vi "test SSL Client Invalid Hostname.vi"(8 "error in (no error)":errorcluster, 11 "TestCase in":refnum<class "test SSL Client.lvclass">) -> (0 "error out":errorcluster, 3 "TestCase out":refnum<class "test SSL Client.lvclass">)   [LabVIEW 2013, in "test SSL Client.lvclass"]
uses:
  test SSL Client.lvclass
  <vilib>/addons/_JKI Toolkits/VI Tester/TestCase.llb/TestCase.lvclass
  SSL_Lib/BIO/BIO.lvclass
  <vilib>/Utility/error.llb/DialogType.ctl
  SSL_Lib/SSL-Context/SSL-Context.lvclass
  SSL_Lib/SSL/SSL.lvclass
  SSL_Lib/SSL/SSL_Mode.ctl
  suite SSL Client/suite SSL Client/SSL Context.vi
  suite SSL Client/suite SSL Client/suite SSL Client.lvclass
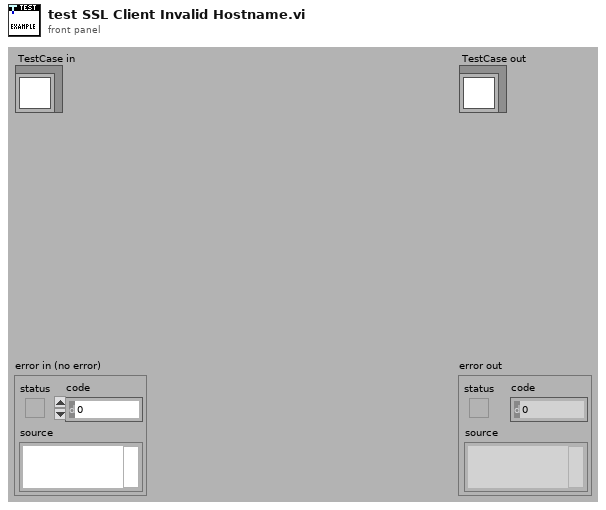
[diagram p1: front panel]
types:
  T1 = typedef "SSL_Lib.lvlib/SSL.lvclass/SSL_Mode.ctl" = i32
  T2 = typedef "DialogType.ctl" = u16
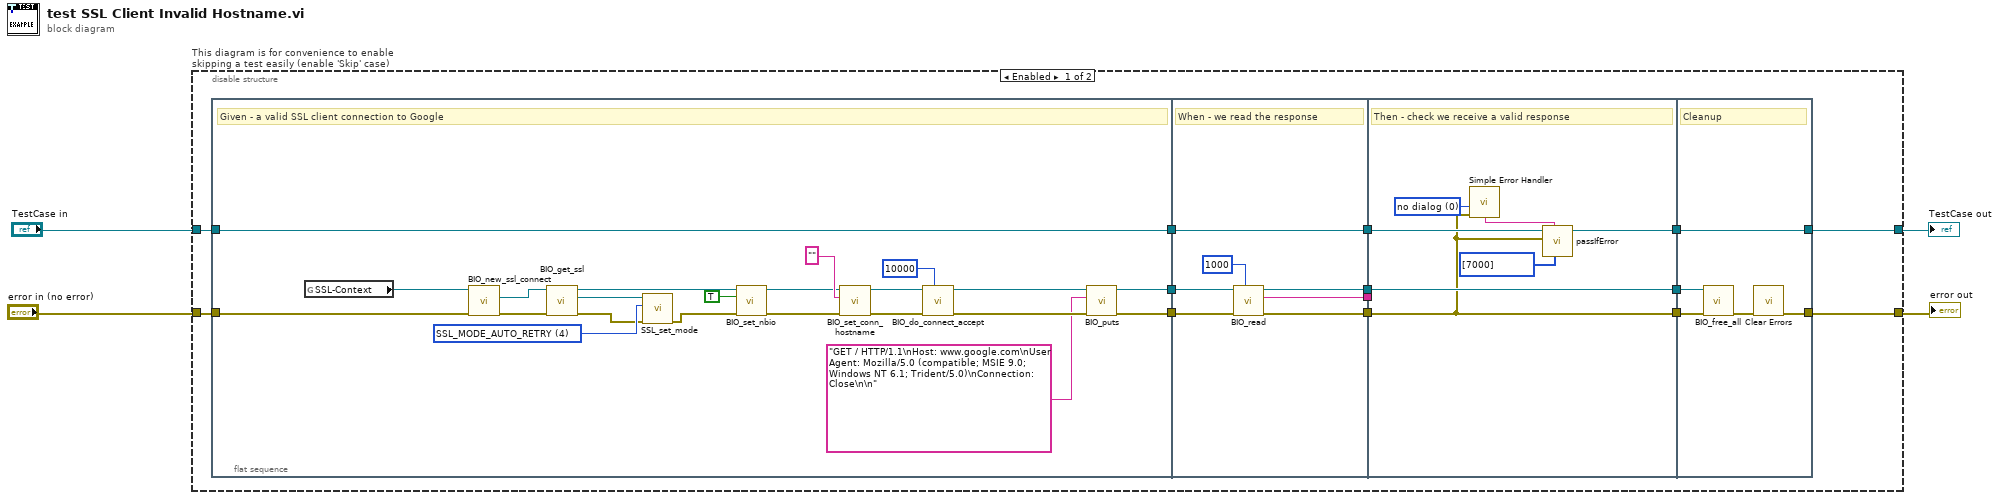
[diagram p0: block diagram]
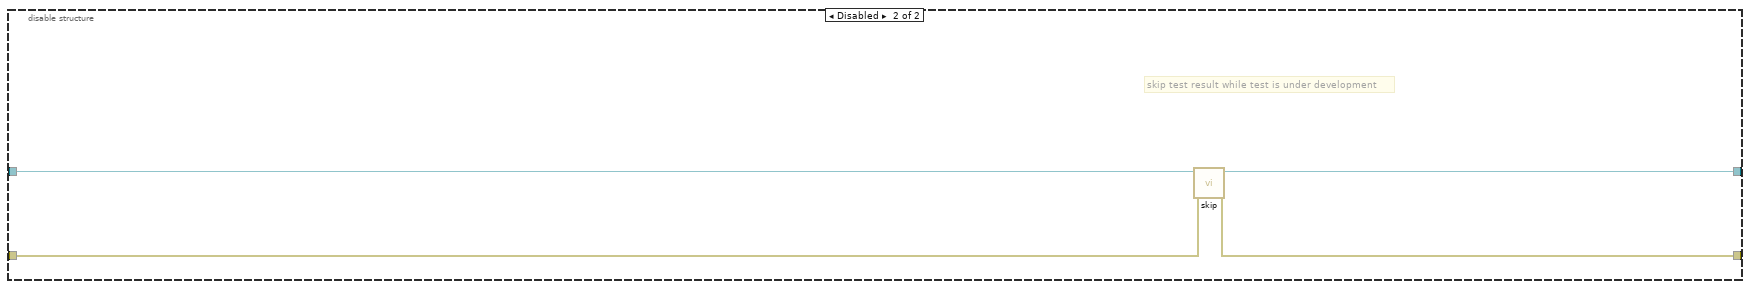
[diagram p2: hidden frame]
diagram:
  n1 = disable-structure "This diagram is for convenience to enable skipping a test easily (enable 'Skip' case)" shown="Enabled" {
    disable-tunnel: "TestCase in" -> [w13 w63]
    disable-tunnel: [w12 w61] -> w1
    disable-tunnel: [w11 w62] -> w3
    disable-tunnel: "error in (no error)" -> [w14 w60]
    frame Enabled {
      n2 = flat-sequence {
        tunnel: w14 -> [w27]
        tunnel: w13 -> [w26]
        tunnel: [w26] -> w18
        tunnel: [w35] -> w10
        tunnel: [w34] -> w9
        tunnel: [w47] -> w17
        tunnel: [w44] -> w16
        tunnel: w18 -> [w47]
        tunnel: w10 -> [w46]
        tunnel: w9 -> [w45]
        tunnel: [w43] -> w8
        tunnel: [w42] -> w7
        tunnel: [w53] -> w15
        tunnel: w17 -> [w54]
        tunnel: w16 -> [w48]
        tunnel: w8 -> [_]
        tunnel: w7 -> [w49]
        tunnel: [w49] -> w6
        tunnel: [w48] -> w5
        tunnel: [w55] -> w11
        tunnel: [w59] -> w12
        tunnel: w15 -> [w59]
        tunnel: w6 -> [w56]
        tunnel: w5 -> [w58]
        frame #0 {
          w29 = T1 4 items=["None"=0, "SSL_MODE_ENABLE_PARTIAL_WRITE"=1, "SSL_MODE_ACCEPT_MOVING_WRITE_BUFFER"=2, "SSL_MODE_AUTO_RETRY"=4, "SSL_MODE_RELEASE_BUFFERS"=16, "SSL_MODE_SEND_FALLBACK_SCSV"=128] ("Mode")
          # "Given - a valid SSL client connection to Google"
          n3 = global read "SSL Context.vi" "SSL-Context"() -> (w25:refnum<class "SSL-Context.lvclass">)
          n4 = call "BIO_new_ssl_connect.vi"("error in (no error)"=w27, "SSL-Context in"=w25) -> ("error out"=w31:errorcluster, "BIO out"=w32:refnum<class "BIO.lvclass">)  [unwired: 7 in, 1 out]
          n5 = call "BIO_get_ssl.vi"("error in (no error)"=w31, "BIO in"=w32) -> ("error out"=w28:errorcluster, "SSL out"=w30:refnum<class "SSL.lvclass">, "BIO out"=w22:refnum<class "BIO.lvclass">)  [unwired: 7 in]
          n6 = call "SSL_set_mode.vi"("error in (no error)"=w28, "Mode"=w29, "SSL in"=w30) -> ("error out"=w23:errorcluster)  [unwired: 7 in, 1 out]
          n7 = call "BIO_set_nbio.vi"("error in (no error)"=w23, "Non-Blocking?"=TRUE, "BIO in"=w22) -> ("error out"=w20:errorcluster, "BIO out"=w21:refnum<class "BIO.lvclass">)  [unwired: 7 in]
          n8 = call "BIO_set_conn_hostname.vi"("error in (no error)"=w20, "Hostname"="", "BIO in"=w21) -> ("error out"=w39:errorcluster, "BIO out"=w33:refnum<class "BIO.lvclass">)  [unwired: 7 in]
          n9 = call "BIO_do_connect_accept.vi"("Timeout (10000ms)"=u32 10000, "error in (no error)"=w39, "BIO in"=w33) -> ("error out"=w37:errorcluster, "BIO out"=w36:refnum<class "BIO.lvclass">)  [unwired: 7 in]
          n10 = call "BIO_puts.vi"("error in (no error)"=w37, "String to write"="GET / HTTP/1.1\nHost: www.google.com\nUser Agent: Mozilla/5.0 (compatible; MSIE 9.0; Windows NT 6.1; Trident/5.0)\nConnection: Close\n\n", "BIO in"=w36) -> ("error out"=w35:errorcluster, "BIO out"=w34:refnum<class "BIO.lvclass">)  [unwired: 7 in]
        }
        frame #1 {
          # "When - we read the response"
          n11 = call "BIO_read.vi"("Timeout (10000ms)"=u32 1000, "error in (no error)"=w46, "BIO in"=w45) -> ("error out"=w44:errorcluster, "String read"=w43:string, "BIO out"=w42:refnum<class "BIO.lvclass">)  [unwired: 6 in]
        }
        frame #2 {
          w50 = T2 0 items=["no dialog", "OK message", "continue or stop message", "OK message + warnings", "continue/stop + warnings"] ("type of dialog (OK msg:1)")
          # "Then - check we receive a valid response"
          n12 = call <vilib>:"Simple Error Handler.vi"("type of dialog (OK msg:1)"=w50, "error in (no error)"=w48) -> ("message"=w51:string)  [unwired: 3 in, 4 out]
          n13 = call-dynamic "passIfError.vi"("passing error codes (default = any error code)"=i32[] [7000], "custom report message (\"\")"=w51, "error"=w48, "TestCase in"=w54) -> ("TestCase out"=w53:refnum<class "test SSL Client.lvclass">)  [unwired: 6 in, 1 out]
        }
        frame #3 {
          # "Cleanup"
          n14 = call "BIO_free_all.vi"("error in (no error)"=w58, "BIO in"=w56) -> ("error out"=w57:errorcluster)  [unwired: 9 in]
          n15 = call <vilib>:"Clear Errors.vi"("error in (no error)"=w57) -> ("error out"=w55:errorcluster)  [unwired: 5 in, 1 out]
        }
      }
    }
    frame Disabled {
      # "skip test result while test is under development"
      n16 = call <vilib>:"skip.vi"("error in (no error)"=w60, "TestCase in"=w63) -> ("error out"=w62:errorcluster, "TestCase out"=w61:refnum<class "test SSL Client.lvclass">)  [unwired: 8 in]
    }
  }
  "error out" <- w3
  "TestCase out" <- w1
